vi "cell_closestToSafeSpace.vi"(6 "manip 1 cell indices":i32[](array[numeric]), 7 "which manipulator":T2(ring), 9 "transform cluster + actuator":T3, 10 "current positions":T1, 11 "current cell locations (px)":dbl[][](array[numeric])) -> (2 "furthest cell index":i32, 3 "closest cell index":i32)   [LabVIEW 2015]
uses:
  <vilib>/Analysis/NI_AALPro.lvlib
  <vilib>/Analysis/_algsub.llb/Real Vector Norm.vi
  <vilib>/Analysis/_algsub.llb/Vector Norm Type.ctl
  pipette cleaning/pressure box/cleaning_soft/controls/actuator_type.ctl
  pipette cleaning/pressure box/cleaning_soft/controls/actuator_cluster.ctl
  machine_vision/coordinate model vis/transform_properties_actuators.ctl
  machine_vision/controls/transform_cluster_actuator.ctl
panel:
  out "cell distances (px)":dbl[](array[numeric])
  # "find cell closest to safe space of manipulator"
  # "returns cell index"
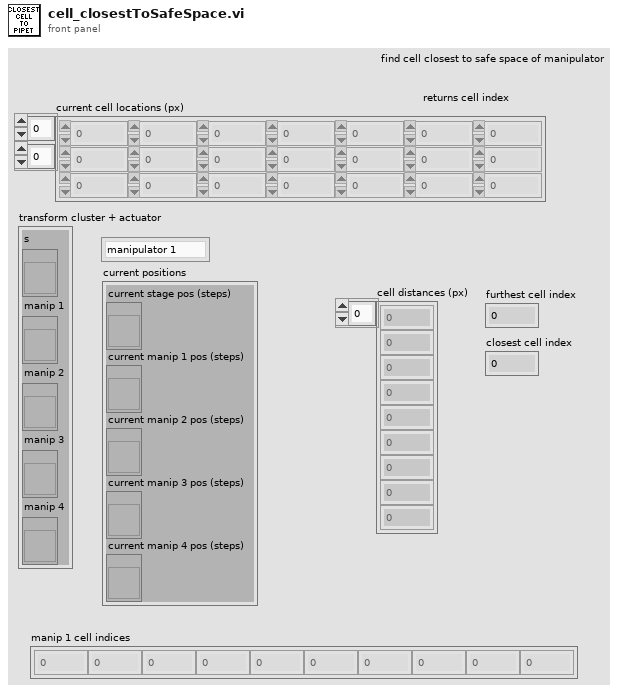
[diagram p1: front panel]
types:
  T1 = cluster{"current stage pos (steps)":refnum<vi>, "current manip 1 pos (steps)":refnum<vi>, "current manip 2 pos (steps)":refnum<vi>, "current manip 3 pos (steps)":refnum<vi>, "current manip 4 pos (steps)":refnum<vi>}
  T2 = enum16{"manipulator 1", "manipulator 2", "manipulator 3", "manipulator 4"}
  T3 = typedef "transform_cluster_actuator.ctl" = cluster{"s":refnum<vi>, "manip 1":refnum<vi>, "manip 2":refnum<vi>, "manip 3":refnum<vi>, "manip 4":refnum<vi>}
  T4 = typedef "transform_properties_actuators.ctl" = cluster{"theta (deg)":dbl, "X sc factor (px/step)":dbl, "Y sc factor (px/step)":dbl, "zero loc (x,y,z)":dbl[], "flip y?":bool, "flip x?":bool, "gamma (deg)":dbl, "flip z?":bool, "Z sc factor (px/step)":dbl, "actuator":T5, "safe space (steps)":i32[]}
  T5 = typedef "actuator_cluster.ctl" = cluster{"Actuator COM":refnum<visa-resource-name>, "Actuator type":T6}
  T6 = typedef "actuator_type.ctl" = enum16{"Scientifica", "Sutter", "Demo", "Off"}
  T7 = typedef "NI_AALPro.lvlib/Vector Norm Type.ctl" = u16
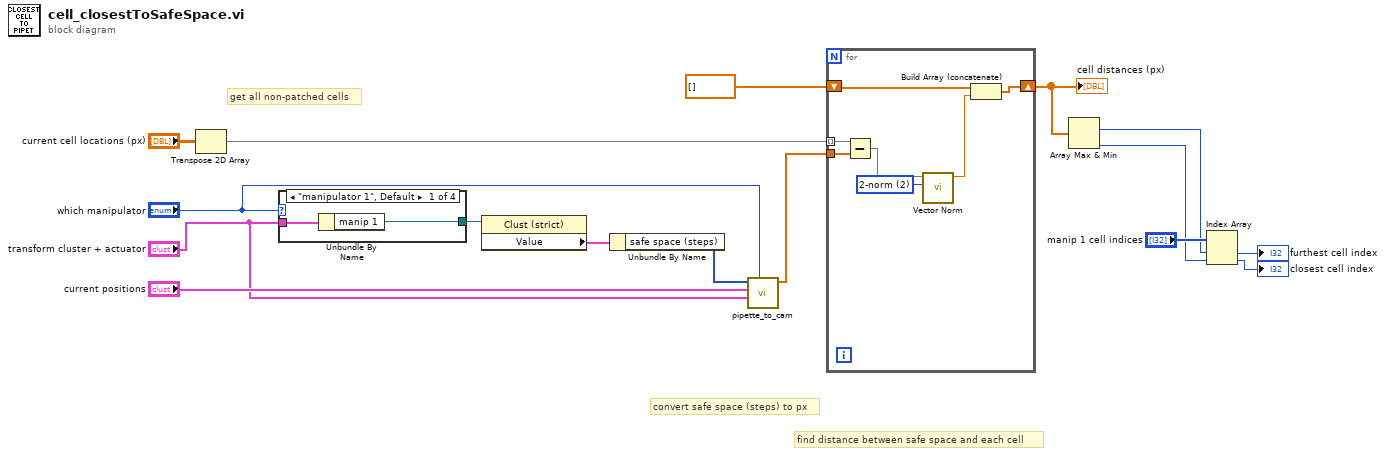
[diagram p0: block diagram]
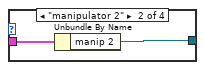
[diagram p2: hidden frame]
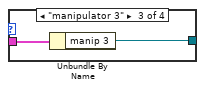
[diagram p3: hidden frame]
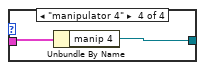
[diagram p4: hidden frame]
diagram:
  # "get all non-patched cells"
  # "find distance between safe space and each cell"
  # "convert safe space (steps) to px"
  n1 = Transpose 2D Array(2D array="current cell locations (px)") -> (transposed array=w1:dbl[][])
  n2 = case shown="\"manipulator 1\", Default" "which manipulator" {
    tunnel: "transform cluster + actuator" -> [w18 w20 w22 w24]
    tunnel: [w17 w19 w21 w23] -> w16
    frame "manipulator 1", Default {
      n3 = Unbundle By Name(w18) -> ("manip 1"=w17:refnum<vi>)
    }
    frame "manipulator 2" {
      n4 = Unbundle By Name(w20) -> ("manip 2"=w19:refnum<vi>)
    }
    frame "manipulator 3" {
      n5 = Unbundle By Name(w22) -> ("manip 3"=w21:refnum<vi>)
    }
    frame "manipulator 4" {
      n6 = Unbundle By Name(w24) -> ("manip 4"=w23:refnum<vi>)
    }
  }
  n7 = property class="Clust (strict)"(reference=w16) -> ("Value"=w15:T4)  [unwired: 1 in, 2 out]
  n8 = Unbundle By Name(w15) -> ("safe space (steps)"=w14:i32[])
  n9 = call "pipette_to_cam.vi"("which manipulator"="which manipulator", "transform cluster + actuator"="transform cluster + actuator", "current positions"="current positions", "pipette position (steps)"=w14) -> ("pipette position (px)"=w10:dbl[])  [unwired: 7 in]
  n10 = for {
    tunnel: w10 -> [w31]
    shift-right: [w27] -> w8
    shift-left: dbl[] [] ("cell distances (px)") -> [w29]
    tunnel: w1 -> [w25] mode=indexing
    w26 = T7 2 items=["1-norm"=1, "2-norm"=2, "Inf-norm"=3, "-Inf-norm"=4, "User Defined"=5] ("norm type")
    n11 = Subtract(x=w25, y=w31) -> (x-y=w30:dbl[])
    n12 = call-poly <vilib>:"Vector Norm.vi"("norm type"=w26, "Input Vector"=w30) -> ("norm"=w28:dbl)  [unwired: 8 in, 1 out]
    n13 = Build Array (concatenate)(w29, w28) -> (w27:dbl[])
  }
  "cell distances (px)" <- w8
  n14 = Array Max & Min(array=w8) -> (max index (indices)=w6:i32, min index (indices)=w5:i32)  [unwired: 2 out]
  n15 = Index Array(array="manip 1 cell indices", index #1=w6, index #2=w5) -> (element #1=→"furthest cell index":i32, element #2=→"closest cell index":i32)
